vi "Configure Laser Output.vi"(8 "error in":errorcluster, 11 "cPAS in":refnum<class "cPAS.lvclass">) -> (0 "error out":errorcluster, 3 "cPAS out":refnum<class "cPAS.lvclass">)   [LabVIEW 2015, in "cPAS.lvclass"]
doc: "Set up the FPGA stuff for operation on the combined PAS/CRDS system deployed during the CalNEX campaign of 2010."
uses:
  cPAS.lvclass
  <vilib>/userdefined/High Color/nirio_resource_hc.ctl
  Reusable/Instrument/Instrument.lvclass/Instrument.ctl
  Reusable/PAS/Main/Controls/Laser Modulation.ctl
  cPAS.lvclass/cPAS.ctl
  Reusable/PAS/Main/PAS.lvclass/PAS.ctl
  Write Speaker Voltage.vi
  Read Speaker Voltage.vi
  Reusable/Instrument/Read Configured.vi
  Reusable/PAS/Main/Read Chirp.vi
  Reusable/PAS/Main/Read Cells.vi
  Reusable/PAS/Cell/Write FPGA_Ctl.vi
  Reusable/PAS/Main/Write Cells.vi
  Reusable/PAS/Main/Set Speaker Switch.vi
  Reusable/PAS/Main/Get Speaker State.vi
  Reusable/PAS/Cell/Read FPGA_Ctl.vi
  <vilib>/FPGAPlugInAG/PXI-7841R/niLvFpga_Open_PXI-7841R.vi
  <vilib>/rvi/interface/common/niFpgaWaitOnOcc.vi
  <vilib>/Utility/error.llb/Error Cluster From Error Code.vi
  <vilib>/rvi/errors/niLvFpgaAdjustHostInterfaceError.vi
  Write FPGA_Ref.vi
  Reusable/PAS/Cell/PAS Cell.lvclass
  <vilib>/rvi/interface/nirviOpenFPGA/nirviOpenFPGA.xnode
  Interface/fpga_ctl.ctl
  FPGA Bitfiles/FPGA Server.lvbitx
  <vilib>/rvi/interface/nirviMethod/nirviMethod.xnode
  <vilib>/rvi/interface/nirviReadWriteControl/nirviReadWriteControl.xnode
  <vilib>/rvi/errors/niLvFpgaMergeErrorWithErrorCode.vi
  <vilib>/FPGAPlugInAG/PXI-7841R/niLvFpga_ConfigureFifo_PXI-7841R.vi
  <vilib>/FPGAPlugInAG/PXI-7841R/niLvFpga_StartFifo_PXI-7841R.vi
  NiFpgaLv.dll
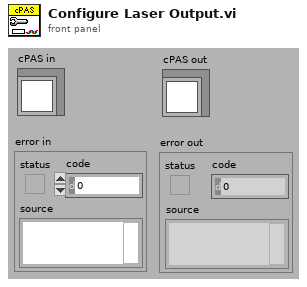
[diagram p1: front panel]
types:
  T1 = cluster{"Ch1":bool, "Ch2":bool, "Ch3":bool, "Ch4":bool, "Ch5":bool}
  T2 = typedef "nirio_resource_hc.ctl" = tag
  T3 = typedef "Laser Modulation.ctl" = enum8{"Sine", "Square"}
  T4 = typedef "fpga_ctl.ctl" = refnum<k20>
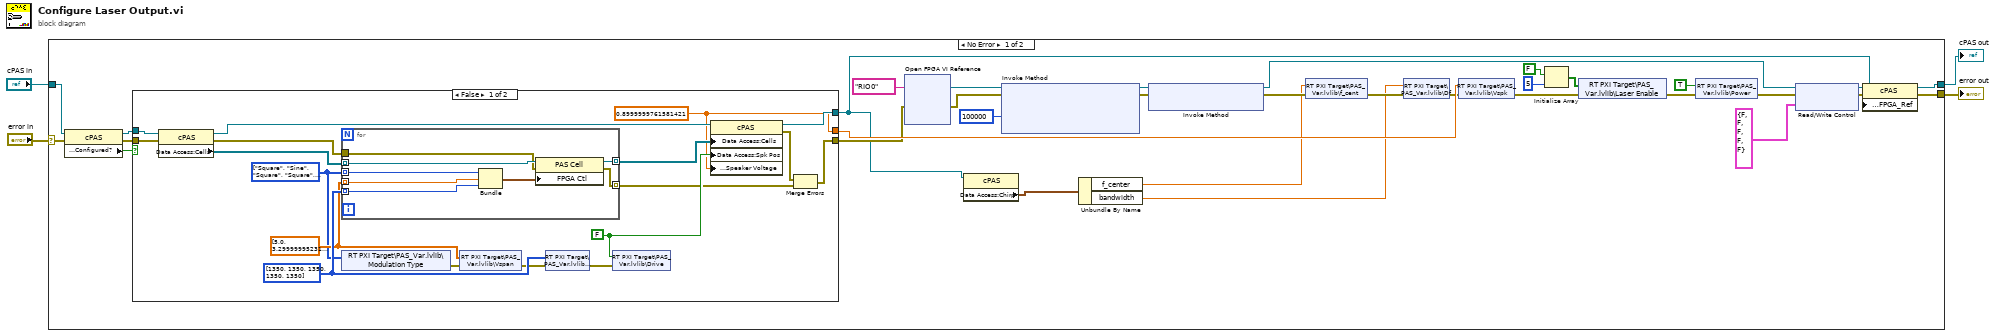
[diagram p0: block diagram]
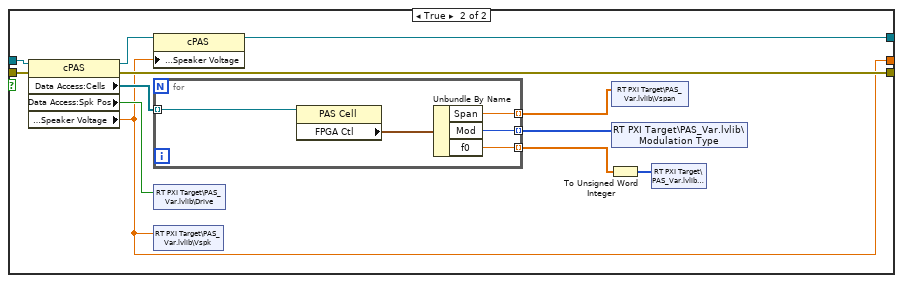
[diagram p2: hidden frame]
diagram:
  n1 = case shown="No Error" "error in" {
    selector: "error in" -> [w33 w82]
    tunnel: [w36 w82] -> w4
    tunnel: [w37 w81] -> w3
    tunnel: "cPAS in" -> [w35 w81]
    frame No Error {
      n2 = property class="cPAS"(reference=w35, error in=w33) -> (reference out=w34:refnum<class "cPAS.lvclass">, error out=w32:errorcluster, "Data Access:Configured?"=w31:bool)
      n3 = case shown="False" w31 {
        tunnel: [w50 w65] -> w8
        tunnel: [w39 w75] -> w20
        tunnel: w34 -> [w55 w73]
        tunnel: w32 -> [w54 w72]
        tunnel: [w38 w64] -> w21
        frame False {
          w43 = T3[] [enum."Square", enum."Sine", enum."Square", enum."Square", enum."Square"] items=["Sine", "Square"] ("array")
          w45 = sgl[] [5.0, 3.3, 5.0, 5.0, 5.0] ("array")
          w47 = u16[] [1350, 1350, 1350, 1350, 1350] ("f0")
          w49 = FALSE
          w38 = sgl 0.9 ("Speake Voltage")
          n4 = property class="cPAS"(reference=w55, error in=w54) -> (reference out=w51:refnum<class "cPAS.lvclass">, error out=w42:errorcluster, "Data Access:Cells"=w53:refnum<class "PAS Cell.lvclass">[])
          n5 = for {
            tunnel: w53 -> [w63] mode=indexing
            tunnel: w45 -> [w62] mode=indexing
            tunnel: w47 -> [w61] mode=indexing
            tunnel: [w60] -> w52 mode=indexing
            tunnel: w43 -> [w59] mode=indexing
            tunnel: w42 -> [w58]
            tunnel: [w57] -> w41 mode=indexing
            n6 = Bundle("ch 1"=w59, "ch 1"=w62, "Cell 1"=w61) -> (w56:cluster{"ch 1":T3, "ch 1":sgl, "Cell 1":u16})  [unwired: 1 in]
            n7 = property class="PAS Cell"(reference=w63, error in=w58, "FPGA Ctl"=w56) -> (reference out=w60:refnum<class "PAS Cell.lvclass">, error out=w57:errorcluster)
          }
          n8 = shared-variable "RT PXI Target\\PAS_Var.lvlib\\Modulation Type"(w43) -> (error out=w44:errorcluster)  [unwired: 1 in]
          n9 = shared-variable "RT PXI Target\\PAS_Var.lvlib\\Vspan"(w45, error in=w44) -> (error out=w46:errorcluster)
          n10 = shared-variable "RT PXI Target\\PAS_Var.lvlib\\f0"(w47, error in=w46) -> (error out=w48:errorcluster)
          n11 = shared-variable "RT PXI Target\\PAS_Var.lvlib\\Drive"(w49, error in=w48) -> ()  [unwired: 1 out]
          n12 = property class="cPAS"(reference=w51, "Data Access:Cells"=w52, "Data Access:Spk Pos"=w49, "Data Access:Speaker Voltage"=w38) -> (reference out=w50:refnum<class "cPAS.lvclass">, error out=w40:errorcluster)  [unwired: 1 in]
          n13 = Merge Errors(w40, w41) -> (w39:errorcluster)
        }
        frame True {
          n14 = property class="cPAS"(reference=w73, error in=w72) -> (reference out=w66:refnum<class "cPAS.lvclass">, error out=w75:errorcluster, "Data Access:Cells"=w74:refnum<class "PAS Cell.lvclass">[], "Data Access:Spk Pos"=w71:bool, "Data Access:Speaker Voltage"=w64:sgl)
          n15 = property class="cPAS"(reference=w66, "Data Access:Speaker Voltage"=w64) -> (reference out=w65:refnum<class "cPAS.lvclass">)  [unwired: 1 in, 1 out]
          n16 = for {
            tunnel: w74 -> [w80] mode=indexing
            tunnel: [w79] -> w69 mode=indexing
            tunnel: [w78] -> w70 mode=indexing
            tunnel: [w77] -> w68 mode=indexing
            n17 = property class="PAS Cell"(reference=w80) -> ("FPGA Ctl"=w76:cluster{"Mod":T3, "Span":sgl, "f0":sgl})  [unwired: 1 in, 2 out]
            n18 = Unbundle By Name(w76) -> ("Span"=w79:sgl, "Mod"=w78:T3, "f0"=w77:sgl)
          }
          n19 = shared-variable "RT PXI Target\\PAS_Var.lvlib\\Drive"(w71) -> ()  [unwired: 1 in, 1 out]
          n20 = shared-variable "RT PXI Target\\PAS_Var.lvlib\\Vspk"(w64) -> ()  [unwired: 1 in, 1 out]
          n21 = To Unsigned Word Integer(number=w68) -> (unsigned 16bit integer=w67:u16[])
          n22 = shared-variable "RT PXI Target\\PAS_Var.lvlib\\Vspan"(w69) -> ()  [unwired: 1 in, 1 out]
          n23 = shared-variable "RT PXI Target\\PAS_Var.lvlib\\Modulation Type"(w70) -> ()  [unwired: 1 in, 1 out]
          n24 = shared-variable "RT PXI Target\\PAS_Var.lvlib\\f0"(w67) -> ()  [unwired: 1 in, 1 out]
        }
      }
      n25 = xnode "Open FPGA VI Reference"("error in"=w20, "resource name"=T2 "RIO0") -> ("FPGA VI Reference Out"=w16:T4, "error out"=w12:errorcluster)
      n26 = property class="cPAS"(reference=w8) -> ("Data Access:Chirp"=w7:cluster{"f_center":dbl, "bandwidth":dbl})  [unwired: 1 in, 2 out]
      n27 = xnode "Invoke Method"("FPGA VI Reference In"=w16, "error in"=w12, "Requested Depth"=u32 100000) -> ("FPGA VI Reference Out"=w13:T4, "error out"=w11:errorcluster)  [unwired: 1 out]
      n28 = Unbundle By Name(w7) -> ("f_center"=w6:dbl, "bandwidth"=w5:dbl)
      n29 = xnode "Invoke Method"("FPGA VI Reference In"=w13, "error in"=w11) -> ("FPGA VI Reference Out"=w9:T4, "error out"=w10:errorcluster)
      n30 = shared-variable "RT PXI Target\\PAS_Var.lvlib\\f_cent"(w6, error in=w10) -> (error out=w19:errorcluster)
      n31 = shared-variable "RT PXI Target\\PAS_Var.lvlib\\Df"(w5, error in=w19) -> (error out=w18:errorcluster)
      n32 = shared-variable "RT PXI Target\\PAS_Var.lvlib\\Vspk"(w21, error in=w18) -> (error out=w17:errorcluster)
      n33 = Initialize Array(FALSE, 5 ("dimension size")) -> (w23:bool[])
      n34 = shared-variable "RT PXI Target\\PAS_Var.lvlib\\Laser Enable"(w23, error in=w17) -> (error out=w22:errorcluster)
      n35 = shared-variable "RT PXI Target\\PAS_Var.lvlib\\Power"(TRUE ("Power"), error in=w22) -> (error out=w27:errorcluster)
      n36 = xnode "Read/Write Control"("FPGA VI Reference In"=w9, "error in"=w27, "iSpk Enable"=T1 {"Ch1"=FALSE, "Ch2"=FALSE, "Ch3"=FALSE, "Ch4"=FALSE, "Ch5"=FALSE}) -> ("FPGA VI Reference Out"=w15:T4, "error out"=w26:errorcluster)
      n37 = property class="cPAS"(reference=w8, error in=w26, "Data Access:FPGA_Ref"=w15) -> (reference out=w37:refnum<class "cPAS.lvclass">, error out=w36:errorcluster)
    }
    frame Error {
    }
  }
  "error out" <- w4
  "cPAS out" <- w3
